vi "format_vars.vi"(9 "UVARS":string[](array[string]), 10 "vVARS":variant, 11 "Var Array":string[][](array[string])) -> (3 "Vals":string[](array[string]))   [LabVIEW 2013]
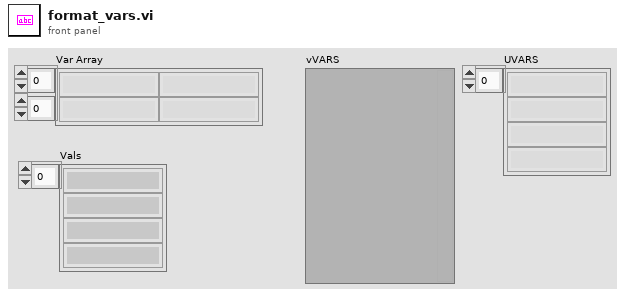
[diagram p1: front panel]
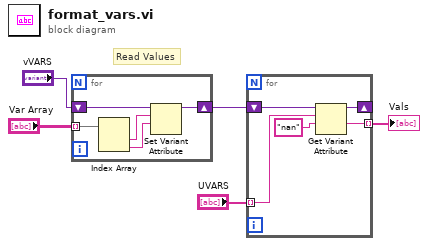
[diagram p0: block diagram]
diagram:
  # "Read Values"
  n1 = for {
    tunnel: "Var Array" -> [w8] mode=indexing
    shift-right: [w9] -> w3
    shift-left: "vVARS" -> [w10]
    n2 = Index Array(array=w8) -> (element #1=w7:string, element #2=w6:string)  [unwired: 2 in]
    n3 = Set Variant Attribute(Variant=w10, name=w7, value=w6) -> (Variant out=w9:variant)  [unwired: 1 in, 2 out]
  }
  n4 = for {
    tunnel: "UVARS" -> [w14] mode=indexing
    shift-right: [w12] -> _
    shift-left: w3 -> [w15]
    tunnel: [w11] -> w2 mode=indexing
    n5 = Get Variant Attribute(Variant=w15, name=w14, default value (empty Variant)="nan") -> (duplicate Variant=w12:variant, value=w11:string)  [unwired: 1 in, 2 out]
  }
  "Vals" <- w2
